vi "Sensor Calibration.vi"(8 "error in":errorcluster, 11 "Sensor Raw SV":refnum<k21>) -> (0 "error out":errorcluster, 2 "New Cal Parameters":T1={"Slope"=62500.0, "Intercept"=-250.0} {"Intercept" format="%.3f"; "Slope" format="%.3f"}, 3 "Update":bool)   [LabVIEW 2018]
uses:
  Controls/Sensor CalPara.ctl
  <vilib>/Analysis/6fits.llb/Curve Fitting Criteria.ctl
  <vilib>/Analysis/NI_AALPro.lvlib
panel:
  out "Old Cal Parameters":T1={"Slope"=62500.0, "Intercept"=-250.0} {"Intercept" format="%.3f"; "Slope" format="%.3f"}
  in  "Data":dbl[][](array[numeric])
  in  "Insert":bool
  in  "Reference Reading (Psig)":dbl
  in  "Raw Reading (A)":dbl
  in  "Cancel":bool
  in  "Update":bool
  out "Residue":dbl
  out "New Intercept":dbl format="%.3f"
  out "New Slope":dbl format="%.3f"
  out "Multiple Plots":cluster{dbl[], "Best Linear Fit":dbl[]}[](graph)
  in  "Calibrate Button":bool
  # "Sensor Calibration"
  # "1. Fill up calibration table"
  # "2. Calibration"
  # "RAW DATA (A)"
  # "REF READING (PSI)"
  # "CAL READING (PSI)"
  # "Differential (%)"
  # "X +"
  # "Notes:\n1. Raw data needs to be averaged on cRIO before send to UI"
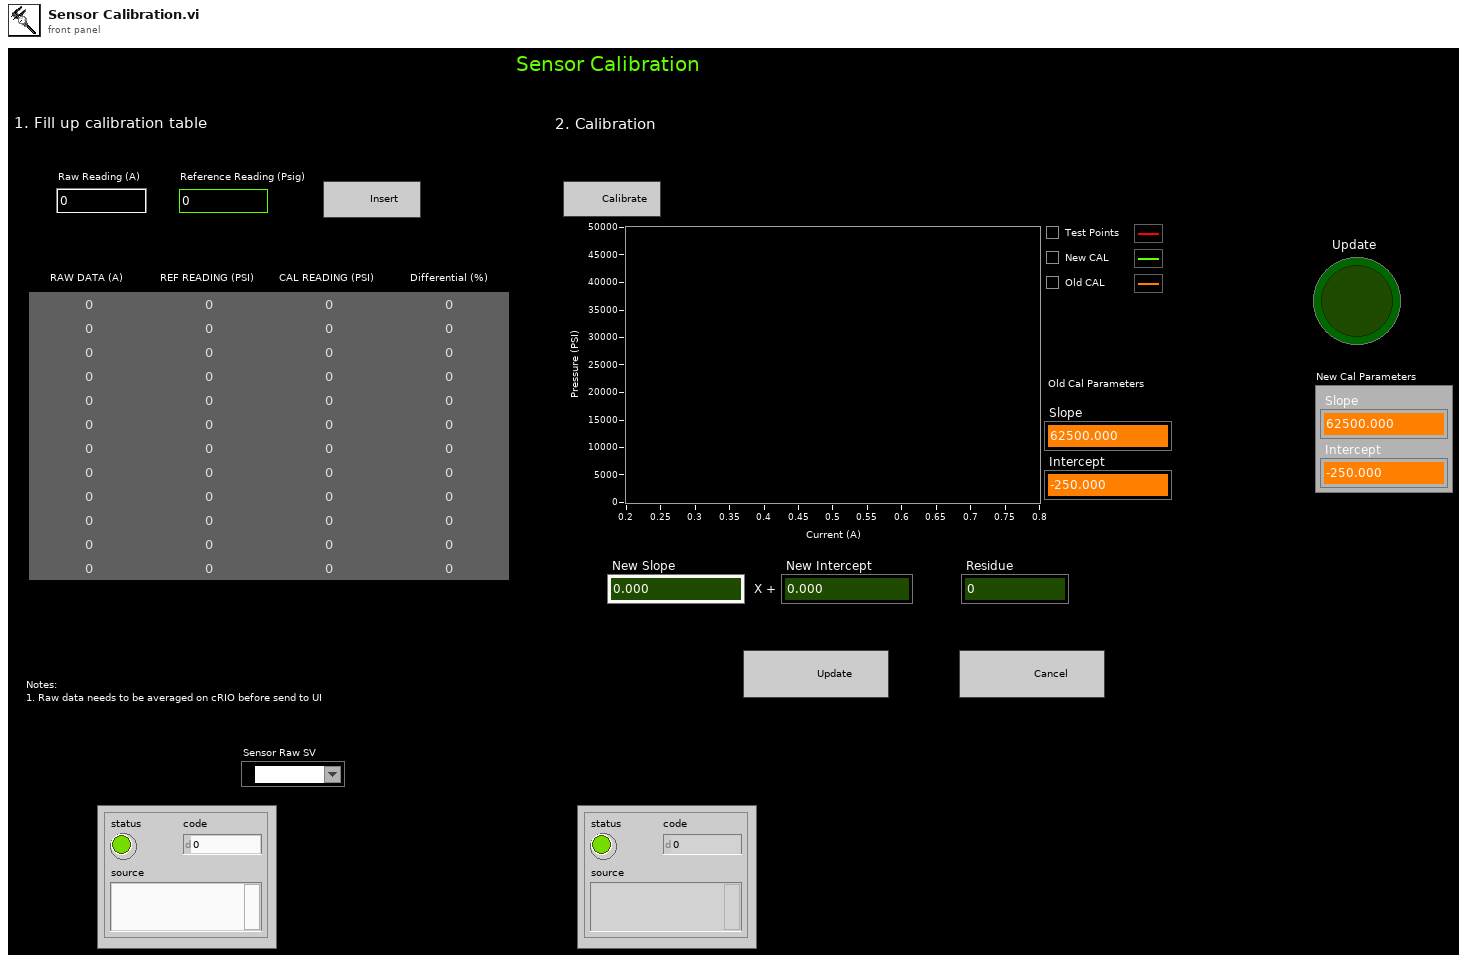
[diagram p1: front panel]
types:
  T1 = typedef "Sensor CalPara.ctl" = cluster{"Slope":dbl, "Intercept":dbl}
  T2 = typedef "NI_AALPro.lvlib/Curve Fitting Criteria.ctl" = u16
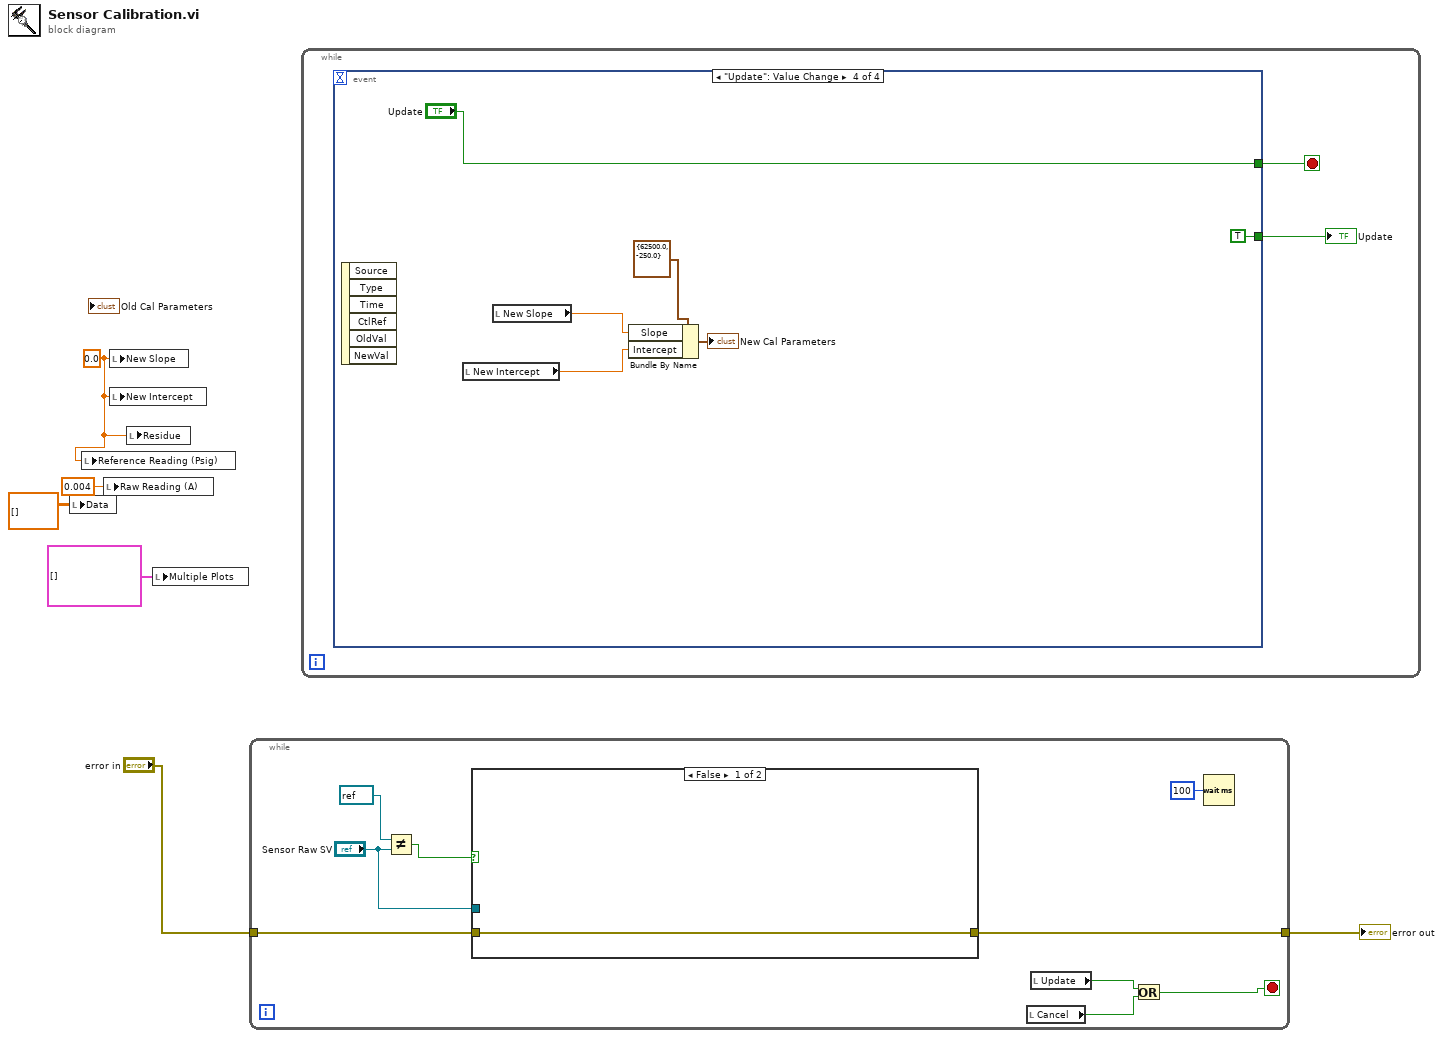
[diagram p0: block diagram]
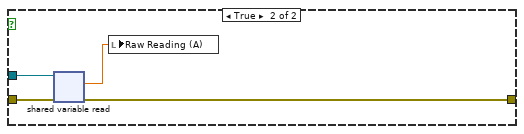
[diagram p2: hidden frame]
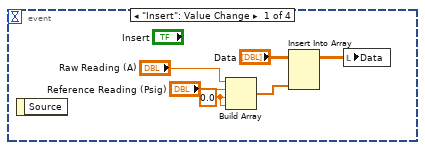
[diagram p3: hidden frame]
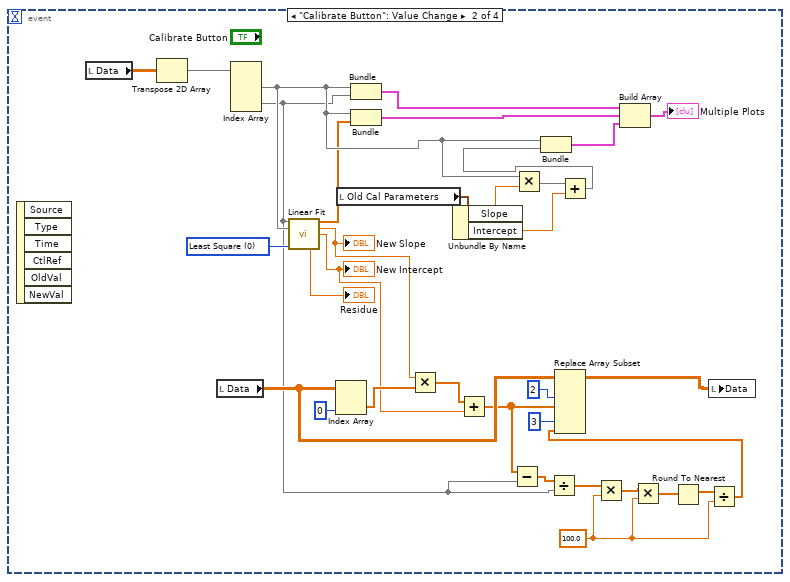
[diagram p4: hidden frame]
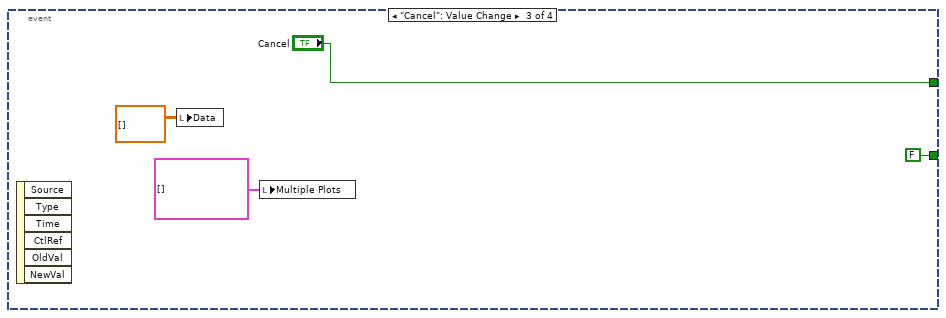
[diagram p5: hidden frame]
diagram:
  w4 = 0.0 ("New Slope")
  n1 = local write "Data"(dbl[][] [] ("Data")) -> ()
  n2 = local write "Reference Reading (Psig)"(w4) -> ()
  n3 = local write "Raw Reading (A)"(0.004 ("Raw Reading (A)")) -> ()
  n4 = local write "New Slope"(w4) -> ()
  n5 = local write "New Intercept"(w4) -> ()
  n6 = local write "Residue"(w4) -> ()
  n7 = local write "Multiple Plots"(cluster{dbl[], "Best Linear Fit":dbl[]}[] [] ("Multiple Plots")) -> ()
  n8 = while {
    tunnel: "error in" -> [w8]
    tunnel: [w7] -> w1
    stop <- w11 stop-if-true
    n9 = Not Equal?(x=refnum<k21> refnum ("Sensor SV"), y="Sensor Raw SV") -> (x != y?=w14:bool)
    n10 = case shown="False" w14 {
      tunnel: "Sensor Raw SV" -> [_ w20]
      tunnel: w8 -> [w16 w19]
      tunnel: [w16 w18] -> w7
      frame False {
      }
      frame True {
        n11 = shared-variable-read(w20, w19) -> (w18:errorcluster, w17:dbl)  [unwired: 2 out]
        n12 = local write "Raw Reading (A)"(w17) -> ()
      }
    }
    n13 = local read "Cancel"() -> (w12:bool)
    n14 = local read "Update"() -> (w13:bool)
    n15 = Or(x=w13, y=w12) -> (x .or. y?=w11:bool)
    n16 = Wait (ms)(milliseconds to wait=u32 100) -> ()  [unwired: 1 out]
  }
  "error out" <- w1
  n17 = while {
    stop <- w22 stop-if-true
    n18 = event shown="[3] \"Update\": Value Change" {
      selector: _ -> [_ _ _ _]
      dyn-events: _ -> [_ _ _ _]
      timeout: _ -> [_ _ _ _]
      tunnel: [_ _ "Cancel" "Update"] -> w22
      tunnel: [_ _ FALSE ("Update") TRUE ("Update")] -> w21
      event "Insert": Value Change {
        w24 = 0.0 ("element")
        n19 = event-data() -> ()  [unwired: 1 in, 1 out]
        n20 = Build Array("Raw Reading (A)", "Reference Reading (Psig)", w24, w24) -> (w26:dbl[])
        n21 = Insert Into Array(array="Data", new element=w26) -> (w25:dbl[][])  [unwired: 2 in]
        n22 = local write "Data"(w25) -> ()
      }
      event "Calibrate Button": Value Change {
        w30 = 100.0
        w61 = T2 0 items=["Least Square", "Least Absolute Residual", "Bisquare"] ("method")
        n23 = event-data() -> ()  [unwired: 1 in, 6 out]
        n24 = local read "Data"() -> (w59:dbl[][])
        n25 = Transpose 2D Array(2D array=w59) -> (transposed array=w60:dbl[][])
        n26 = local read "Data"() -> (w49:dbl[][])
        n27 = Index Array(array=w60) -> (element #1=w46:dbl[], element #2=w34:dbl[])  [unwired: 4 in]
        n28 = call <vilib>:"Linear Fit.vi"("Y"=w34, "X"=w46, "method"=w61) -> ("Best Linear Fit"=w36:dbl[], "slope"=w52:dbl, "intercept"=w50:dbl, "residue"=→"Residue":dbl)  [unwired: 8 in, 1 out]
        "New Slope" <- w52
        "New Intercept" <- w50
        n29 = Index Array(array=w49, index (col)=0 ("disabled index (col)")) -> (element=w53:dbl[])  [unwired: 1 in]
        n30 = local read "Old Cal Parameters"() -> (w42:T1)
        n31 = Bundle(w46, w34) -> (w57:cluster{dbl[], dbl[]})  [unwired: 1 in]
        n32 = Bundle(w46, "Best Linear Fit"=w36) -> (w56:cluster{dbl[], "Best Linear Fit":dbl[]})  [unwired: 1 in]
        n33 = Multiply(x=w52, y=w53) -> (x*y=w51:dbl[])
        n34 = Unbundle By Name(w42) -> ("Slope"=w41:dbl, "Intercept"=w40:dbl)
        n35 = Add(x=w51, y=w50) -> (x+y=w38:dbl[])
        n36 = Subtract(x=w38, y=w34) -> (x-y=w37:dbl[])
        n37 = Multiply(x=w46, y=w41) -> (x*y=w45:dbl[])
        n38 = Divide(x=w37, y=w34) -> (x/y=w35:dbl[])
        n39 = Add(x=w45, y=w40) -> (x+y=w44:dbl[])
        n40 = Bundle(w46, w44) -> (w43:cluster{dbl[], dbl[]})  [unwired: 1 in]
        n41 = Multiply(x=w35, y=w30) -> (x*y=w33:dbl[])
        n42 = Build Array(w57, w56, w43) -> (→"Multiple Plots":cluster{dbl[], "Best Linear Fit":dbl[]}[])
        n43 = Multiply(x=w33, y=w30) -> (x*y=w32:dbl[])
        n44 = Round To Nearest(number=w32) -> (nearest integer value=w31:dbl[])
        n45 = Divide(x=w31, y=w30) -> (x/y=w29:dbl[])
        n46 = Replace Array Subset(array=w49, new element #1=w38, index (col) #1=2 ("disabled index (col)"), new element #2=w29, index (col) #2=3 ("disabled index (row)")) -> (w47:dbl[][])  [unwired: 2 in]
        n47 = local write "Data"(w47) -> ()
      }
      event "Cancel": Value Change {
        n48 = event-data() -> ()  [unwired: 1 in, 6 out]
        n49 = local write "Data"(dbl[][] [] ("Data")) -> ()
        n50 = local write "Multiple Plots"(cluster{dbl[], "Best Linear Fit":dbl[]}[] [] ("Multiple Plots")) -> ()
      }
      event "Update": Value Change {
        n51 = event-data() -> ()  [unwired: 1 in, 6 out]
        n52 = local read "New Intercept"() -> (w69:dbl)
        n53 = local read "New Slope"() -> (w70:dbl)
        n54 = Bundle By Name(cluster=T1 {"Slope"=62500.0, "Intercept"=-250.0} ("Sensor CalPara"), "Slope"=w70, "Intercept"=w69) -> (→"New Cal Parameters":T1)
      }
    }
    "Update" <- w21
  }
